vi "CameraSettings.vi"(0 "Région d'intérêt":i32(ring) items=["2.6\" x 2.6\"", "5.2\" x 5.2\"", "7.7\" x 7.7\"", "10.3\" x 10.3\"", "12.9\" x 12.9\"", "20.6\" x 20.6\""], 1 "ROIStrings":string[](array[string]), 5 "Gain EM":u16(slide) max=3500 step=10 scale=0.0..3500.0, 7 "Refroidissement":u16(ring) items=["Désactivé", "Activé", "Activé & Profond", "Désactivé (sans fan)", "Activé (sans fan)", "Activé & Profond (sans fan)"], 9 "Binning":u16(ring) items=["Binning 1 x 1"=1, "Binning 2 x 2"=2, "Binning 4 x 4"=4, "Binning 5 x 5"=5], 11 "FPS":dbl=0.2 caption="Image retournée par seconde" min=0.2 max=10.0 step=0.1 format="%.1f") -> (4 "Apply Changes":bool, 6 "Cooling_OUT":u16, 8 "Gain_OUT":u16, 10 "Binning_OUT":u16(ring) items=["Binning 1 x 1"=1, "Binning 2 x 2"=2, "Binning 4 x 4"=4, "Binning 5 x 5"=5], 14 "ROISize_OUT":i32, 15 "FPS_OUT":dbl=0.1 caption="Images retournée par secondes" min=0.1 max=30.0 step=1.0 format="%.1g")   [LabVIEW 2019]
panel:
  in  "GainON":bool
  in  "GainOFF":bool
  in  "Default":bool
  in  "cancel":bool
  in  "accept":bool
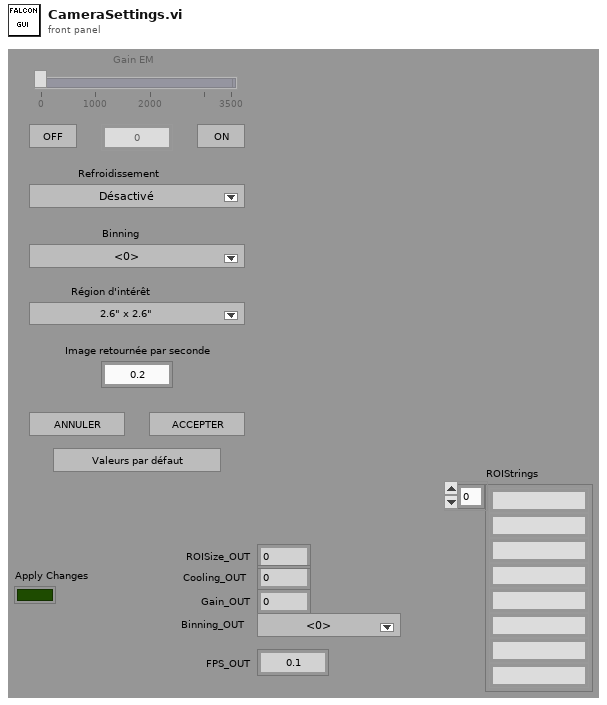
[diagram p1: front panel]
types:
  T1 = enum8{"Enabled", "Disabled", "Disabled and Grayed Out"}
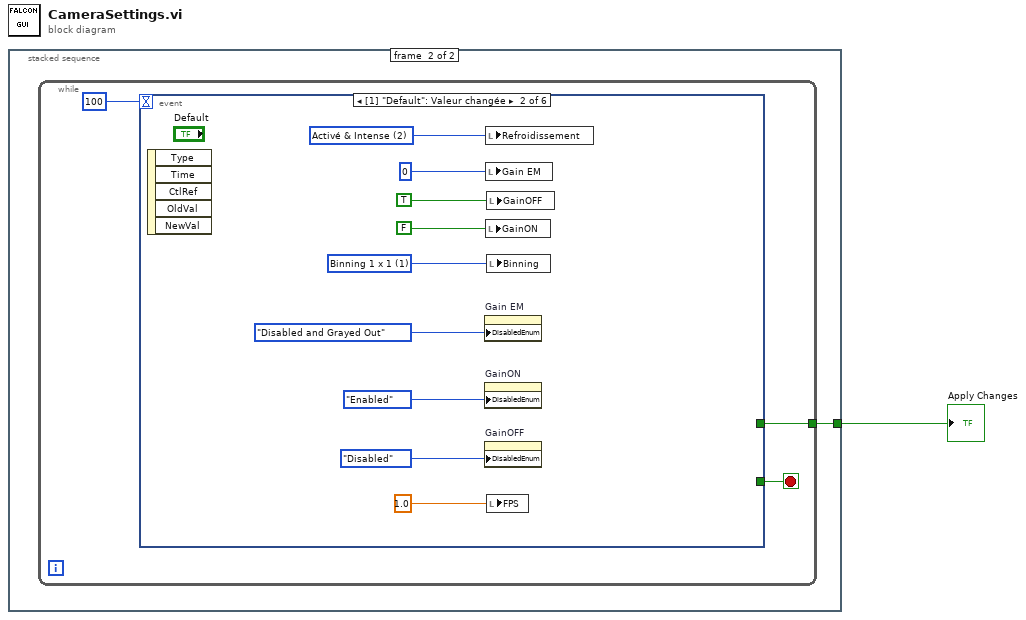
[diagram p0: block diagram]
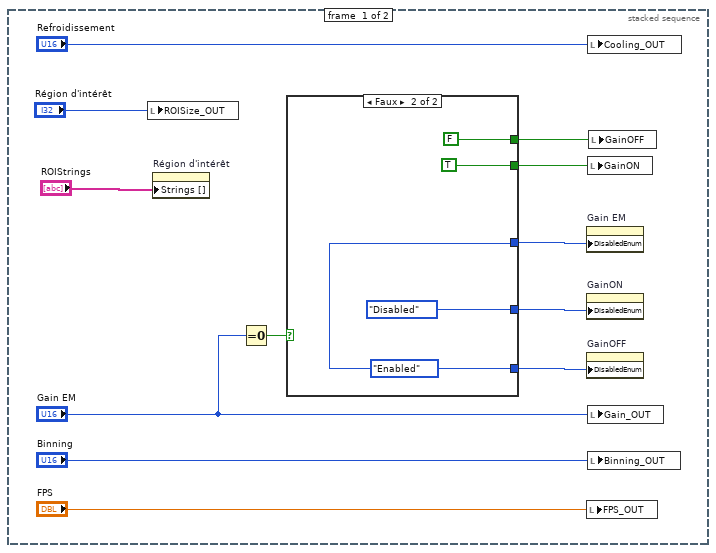
[diagram p2: hidden frame]
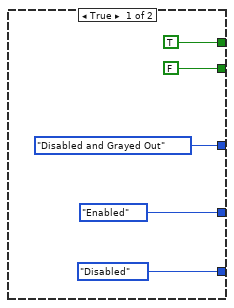
[diagram p3: hidden frame]
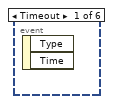
[diagram p4: hidden frame]
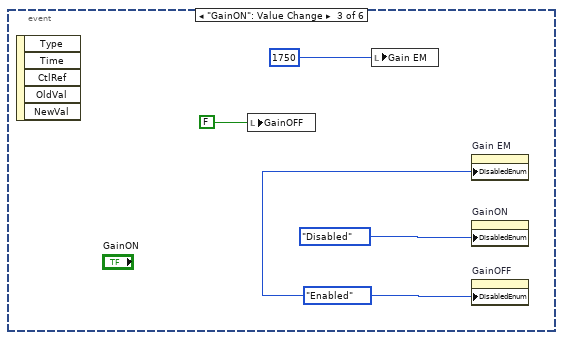
[diagram p5: hidden frame]
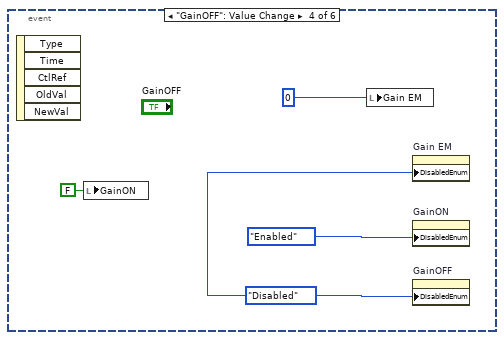
[diagram p6: hidden frame]
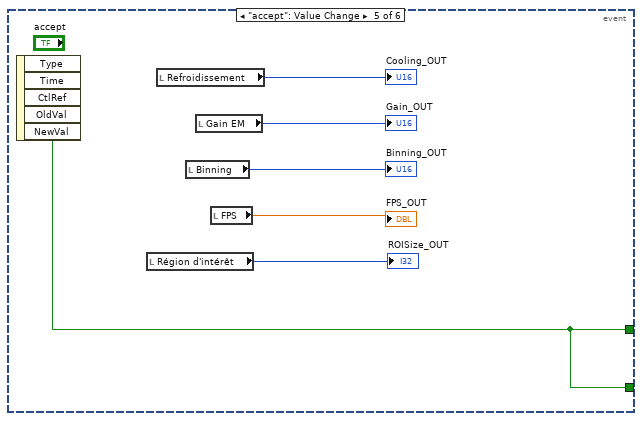
[diagram p7: hidden frame]
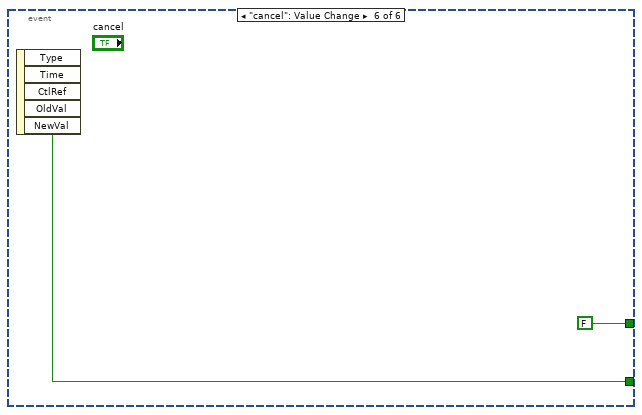
[diagram p8: hidden frame]
diagram:
  n1 = stacked-sequence {
    tunnel: [_ w23] -> w1
    frame #0 {
      n2 = local write "ROISize_OUT"("Région d'intérêt") -> ()
      n3 = property on="Région d'intérêt" class="MDér (strict)"("Strings []"="ROIStrings") -> ()  [unwired: 2 in, 2 out]
      n4 = Equal To 0?(x="Gain EM") -> (x = 0?=w11:bool)
      n5 = case shown="Faux" w11 {
        tunnel: [T1."Enabled" ("Disabled") T1."Disabled" ("Disabled")] -> w9
        tunnel: [T1."Disabled" ("Disabled") w21] -> w8
        tunnel: [T1."Disabled and Grayed Out" ("Disabled") w21] -> w7
        tunnel: [FALSE TRUE] -> w6
        tunnel: [TRUE FALSE] -> w5
        frame True {
        }
        frame False {
          w21 = T1."Enabled" ("Disabled")
        }
      }
      n6 = property on="Gain EM" class="Gliss (strict)"("DisabledEnum"=w7) -> ()  [unwired: 2 in, 2 out]
      n7 = property on="GainON" class="Bool (strict)"("DisabledEnum"=w9) -> ()  [unwired: 2 in, 2 out]
      n8 = property on="GainOFF" class="Bool (strict)"("DisabledEnum"=w8) -> ()  [unwired: 2 in, 2 out]
      n9 = local write "FPS_OUT"("FPS") -> ()
      n10 = local write "Cooling_OUT"("Refroidissement") -> ()
      n11 = local write "GainON"(w6) -> ()
      n12 = local write "Gain_OUT"("Gain EM") -> ()
      n13 = local write "Binning_OUT"("Binning") -> ()
      n14 = local write "GainOFF"(w5) -> ()
    }
    frame #1 {
      n15 = while {
        tunnel: [w25] -> w23
        stop <- w26 stop-if-true
        n16 = event shown="[1] \"Default\": Valeur changée" {
          selector: _ -> [_ _ _ _ _ _]
          dyn-events: _ -> [_ _ _ _ _ _]
          timeout: 100 -> [_ _ _ _ _ _]
          tunnel: [_ _ _ _ w49 w51] -> w26
          tunnel: [_ _ _ _ w49 FALSE ("accept")] -> w25
          event Timeout {
            n17 = event-data() -> ()  [unwired: 1 in, 2 out]
          }
          event "Default": Value Change {
            w34 = u16 2 items=["Désactivé", "Activé", "Activé & Intense"] ("Refroidissement")
            w35 = u16 1 items=["Binning 1 x 1"=1, "Binning 2 x 2"=2, "Binning 4 x 4"=4, "Binning 5 x 5"=5] ("Binning")
            n18 = event-data() -> ()  [unwired: 1 in, 5 out]
            n19 = property on="Gain EM" class="Gliss (strict)"("DisabledEnum"=T1."Disabled and Grayed Out" ("Disabled")) -> ()  [unwired: 2 in, 2 out]
            n20 = property on="GainON" class="Bool (strict)"("DisabledEnum"=T1."Enabled" ("Disabled")) -> ()  [unwired: 2 in, 2 out]
            n21 = property on="GainOFF" class="Bool (strict)"("DisabledEnum"=T1."Disabled" ("Disabled")) -> ()  [unwired: 2 in, 2 out]
            n22 = local write "Refroidissement"(w34) -> ()
            n23 = local write "Gain EM"(u16 0 ("Gain EM")) -> ()
            n24 = local write "GainON"(FALSE ("GainON")) -> ()
            n25 = local write "GainOFF"(TRUE ("GainOFF")) -> ()
            n26 = local write "Binning"(w35) -> ()
            n27 = local write "FPS"(1.0 ("FPS")) -> ()
          }
          event "GainON": Value Change {
            w39 = T1."Enabled" ("Disabled")
            n28 = event-data() -> ()  [unwired: 1 in, 5 out]
            n29 = local write "GainOFF"(FALSE ("GainOFF")) -> ()
            n30 = local write "Gain EM"(u16 1750 ("Gain EM")) -> ()
            n31 = property on="Gain EM" class="Gliss (strict)"("DisabledEnum"=w39) -> ()  [unwired: 2 in, 2 out]
            n32 = property on="GainON" class="Bool (strict)"("DisabledEnum"=T1."Disabled" ("Disabled")) -> ()  [unwired: 2 in, 2 out]
            n33 = property on="GainOFF" class="Bool (strict)"("DisabledEnum"=w39) -> ()  [unwired: 2 in, 2 out]
          }
          event "GainOFF": Value Change {
            w43 = T1."Disabled" ("Disabled")
            n34 = event-data() -> ()  [unwired: 1 in, 5 out]
            n35 = local write "GainON"(FALSE ("GainON")) -> ()
            n36 = local write "Gain EM"(u16 0 ("Gain EM")) -> ()
            n37 = property on="Gain EM" class="Gliss (strict)"("DisabledEnum"=w43) -> ()  [unwired: 2 in, 2 out]
            n38 = property on="GainON" class="Bool (strict)"("DisabledEnum"=T1."Enabled" ("Disabled")) -> ()  [unwired: 2 in, 2 out]
            n39 = property on="GainOFF" class="Bool (strict)"("DisabledEnum"=w43) -> ()  [unwired: 2 in, 2 out]
          }
          event "accept": Value Change {
            n40 = event-data() -> ("NewVal"=w49:bool)  [unwired: 1 in, 4 out]
            n41 = local read "Région d'intérêt"() -> (→"ROISize_OUT":i32)
            n42 = local read "Refroidissement"() -> (→"Cooling_OUT":u16)
            n43 = local read "Binning"() -> (→"Binning_OUT":u16)
            n44 = local read "Gain EM"() -> (→"Gain_OUT":u16)
            n45 = local read "FPS"() -> (→"FPS_OUT":dbl)
          }
          event "cancel": Value Change {
            n46 = event-data() -> ("NewVal"=w51:bool)  [unwired: 1 in, 4 out]
          }
        }
      }
    }
  }
  "Apply Changes" <- w1
